vi "Tab find.vi"(0 "TabCtl Refnum":refnum<vi>, 5 "VI Refnum":refnum<vi>, 11 "error in (no error)":errorcluster) -> (4 "SP ref out":refnum<vi>, 8 "Boolean":bool, 15 "error out":errorcluster)   [LabVIEW 2016, in "Drona Path obtn.lvlib"]
doc: "This VI is called when a tab is present in a VI whose control's drona path is to be found"
uses:
  Drona Path obtn.lvlib
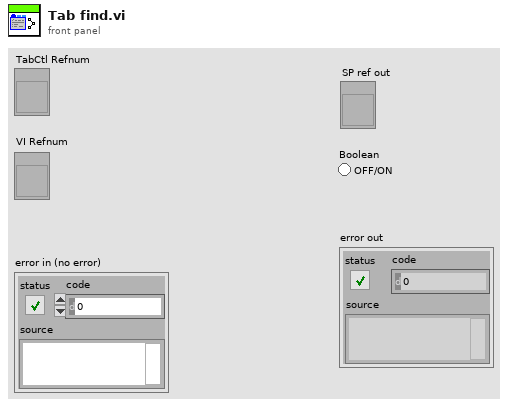
[diagram p1: front panel]
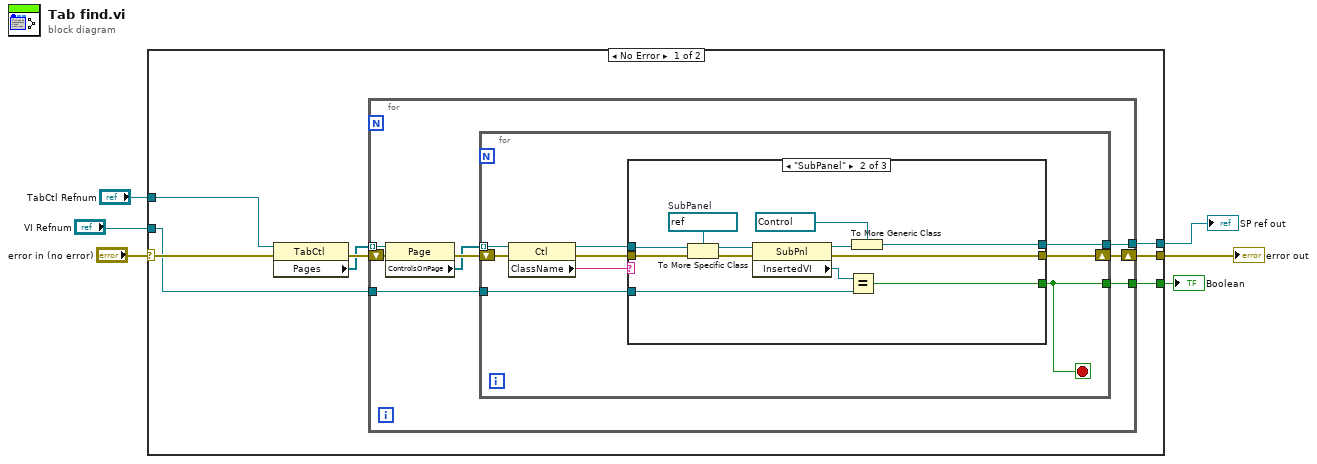
[diagram p0: block diagram]
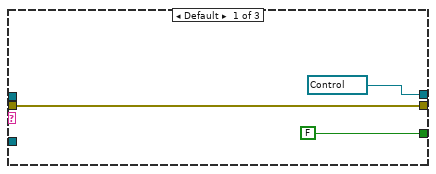
[diagram p2: hidden frame]
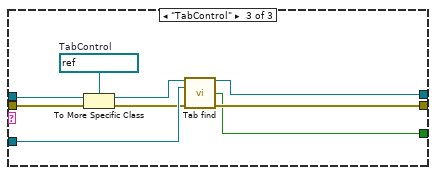
[diagram p3: hidden frame]
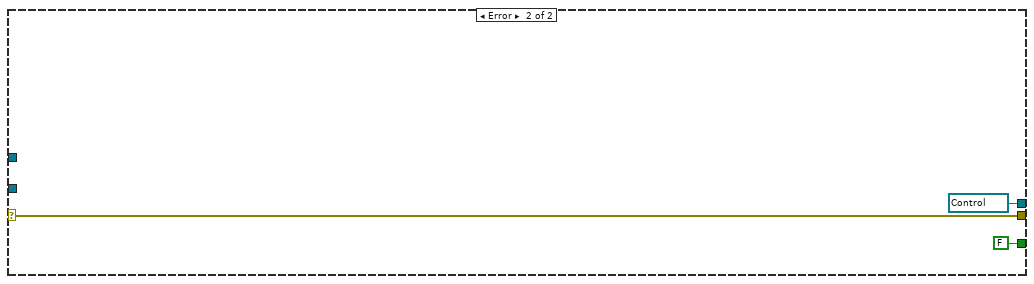
[diagram p4: hidden frame]
diagram:
  n1 = case shown="No Error" "error in (no error)" {
    selector: "error in (no error)" -> [w14 w58]
    tunnel: [w11 w58] -> w5
    tunnel: "VI Refnum" -> [w7 _]
    tunnel: "TabCtl Refnum" -> [w12 _]
    tunnel: [w9 FALSE] -> w3
    tunnel: [w8 refnum<vi> refnum ("SP ref out")] -> w2
    frame No Error {
      n2 = property class="TabCtl"(reference=w12, error in=w14) -> (error out=w13:errorcluster, "Pages"=w10:refnum<vi>[])  [unwired: 1 out]
      n3 = for {
        tunnel: w10 -> [w21] mode=indexing
        shift-right: [w19] -> w11
        shift-left: w13 -> [w22]
        tunnel: w7 -> [w17]
        tunnel: [w16] -> w8
        tunnel: [w15] -> w9
        n4 = property class="Page"(reference=w21, error in=w22) -> (error out=w20:errorcluster, "ControlsOnPage"=w18:refnum<vi>[])  [unwired: 1 out]
        n5 = for {
          shift-right: [w25] -> w19
          shift-left: w20 -> [w28]
          tunnel: w18 -> [w23] mode=indexing
          tunnel: w17 -> [w27]
          tunnel: [w26] -> w16
          tunnel: [w24] -> w15
          stop <- w24 stop-if-true
          n6 = property class="Ctl"(reference=w23, error in=w28) -> (reference out=w31:refnum<vi>, error out=w30:errorcluster, "ClassName"=w29:string)
          n7 = case shown="\"SubPanel\"" w29 {
            tunnel: w30 -> [w34 w46 w55]
            tunnel: [w34 w38 w54] -> w25
            tunnel: w31 -> [_ w44 w51]
            tunnel: w27 -> [_ w40 w53]
            tunnel: [FALSE w39 w47] -> w24
            tunnel: [refnum<vi> refnum ("SP ref out") w35 w48] -> w26
            frame Default {
            }
            frame "SubPanel" {
              w42 = refnum<vi> refnum  # SubPanel
              n8 = To More Specific Class(target class=w42, reference=w44, error in=w46) -> (specific class reference=w43:refnum<vi>, error out=w45:errorcluster)
              n9 = property class="SubPnl"(reference=w43, error in=w45) -> (reference out=w37:refnum<vi>, error out=w38:errorcluster, "InsertedVI"=w41:refnum<vi>)
              n10 = Equal?(x=w41, y=w40) -> (x = y?=w39:bool)
              n11 = To More Generic Class(target class=refnum<vi> refnum ("Ctl Refnum"), reference=w37) -> (generic class reference=w35:refnum<vi>)
            }
            frame "TabControl" {
              w50 = refnum<vi> refnum  # TabControl
              n12 = To More Specific Class(target class=w50, reference=w51, error in=w55) -> (specific class reference=w49:refnum<vi>, error out=w52:errorcluster)
              n13 = call "Tab find.vi"("TabCtl Refnum"=w49, "VI Refnum"=w53, "error in (no error)"=w52) -> ("SP ref out"=w48:refnum<vi>, "Boolean"=w47:bool, "error out"=w54:errorcluster)  [unwired: 10 in]
            }
          }
        }
      }
    }
    frame Error {
    }
  }
  "error out" <- w5
  "Boolean" <- w3
  "SP ref out" <- w2
